vi "TOSA_MCS_Switch_Ray.vi"() -> ()   [LabVIEW 2012]
uses:
  <vilib>/DAQmx/create/channels.llb/DAQmx Create Channel (CO-Pulse Generation-Ticks).vi
  <vilib>/DAQmx/configure/timing.llb/DAQmx Timing (Implicit).vi
  <resource>/objmgr/daqmx.rc
  <vilib>/DAQmx/create/channels.llb/DAQmx Create Channel (DO-Digital Output).vi
panel:
  out "Error Out":errorcluster
  in  "stop 3":bool
  in  "Error In 3":errorcluster
  out "Error Out 3":errorcluster
  in  "Error In":errorcluster
  in  "Stop":bool
  in  "pulse count":u32=150 min=4 max=9000 step=2
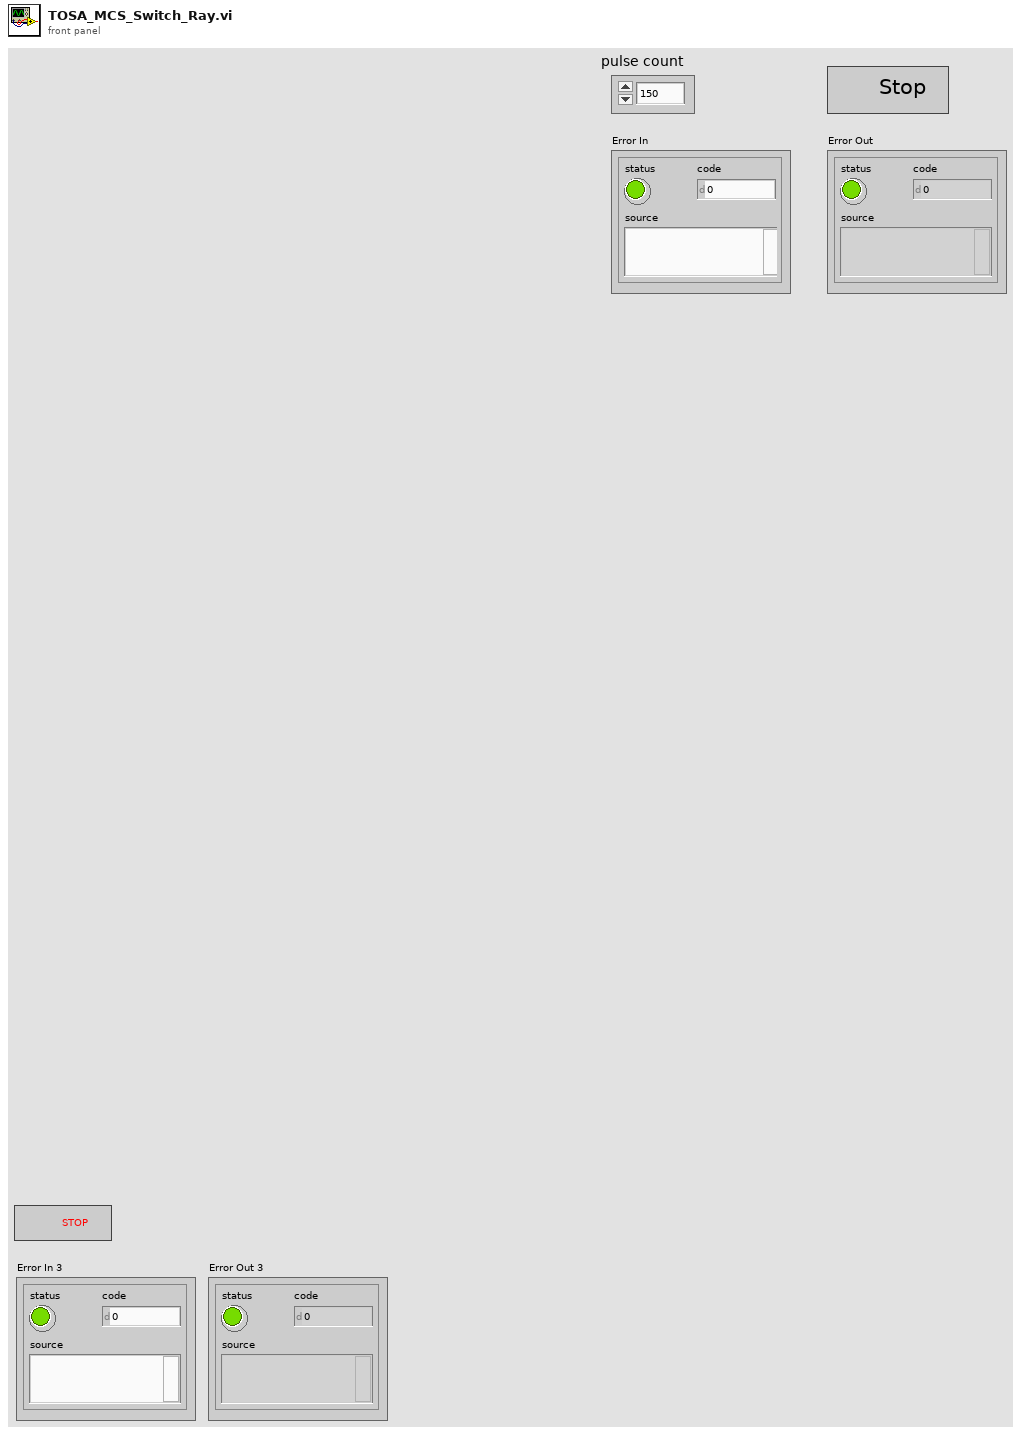
[diagram p1: front panel]
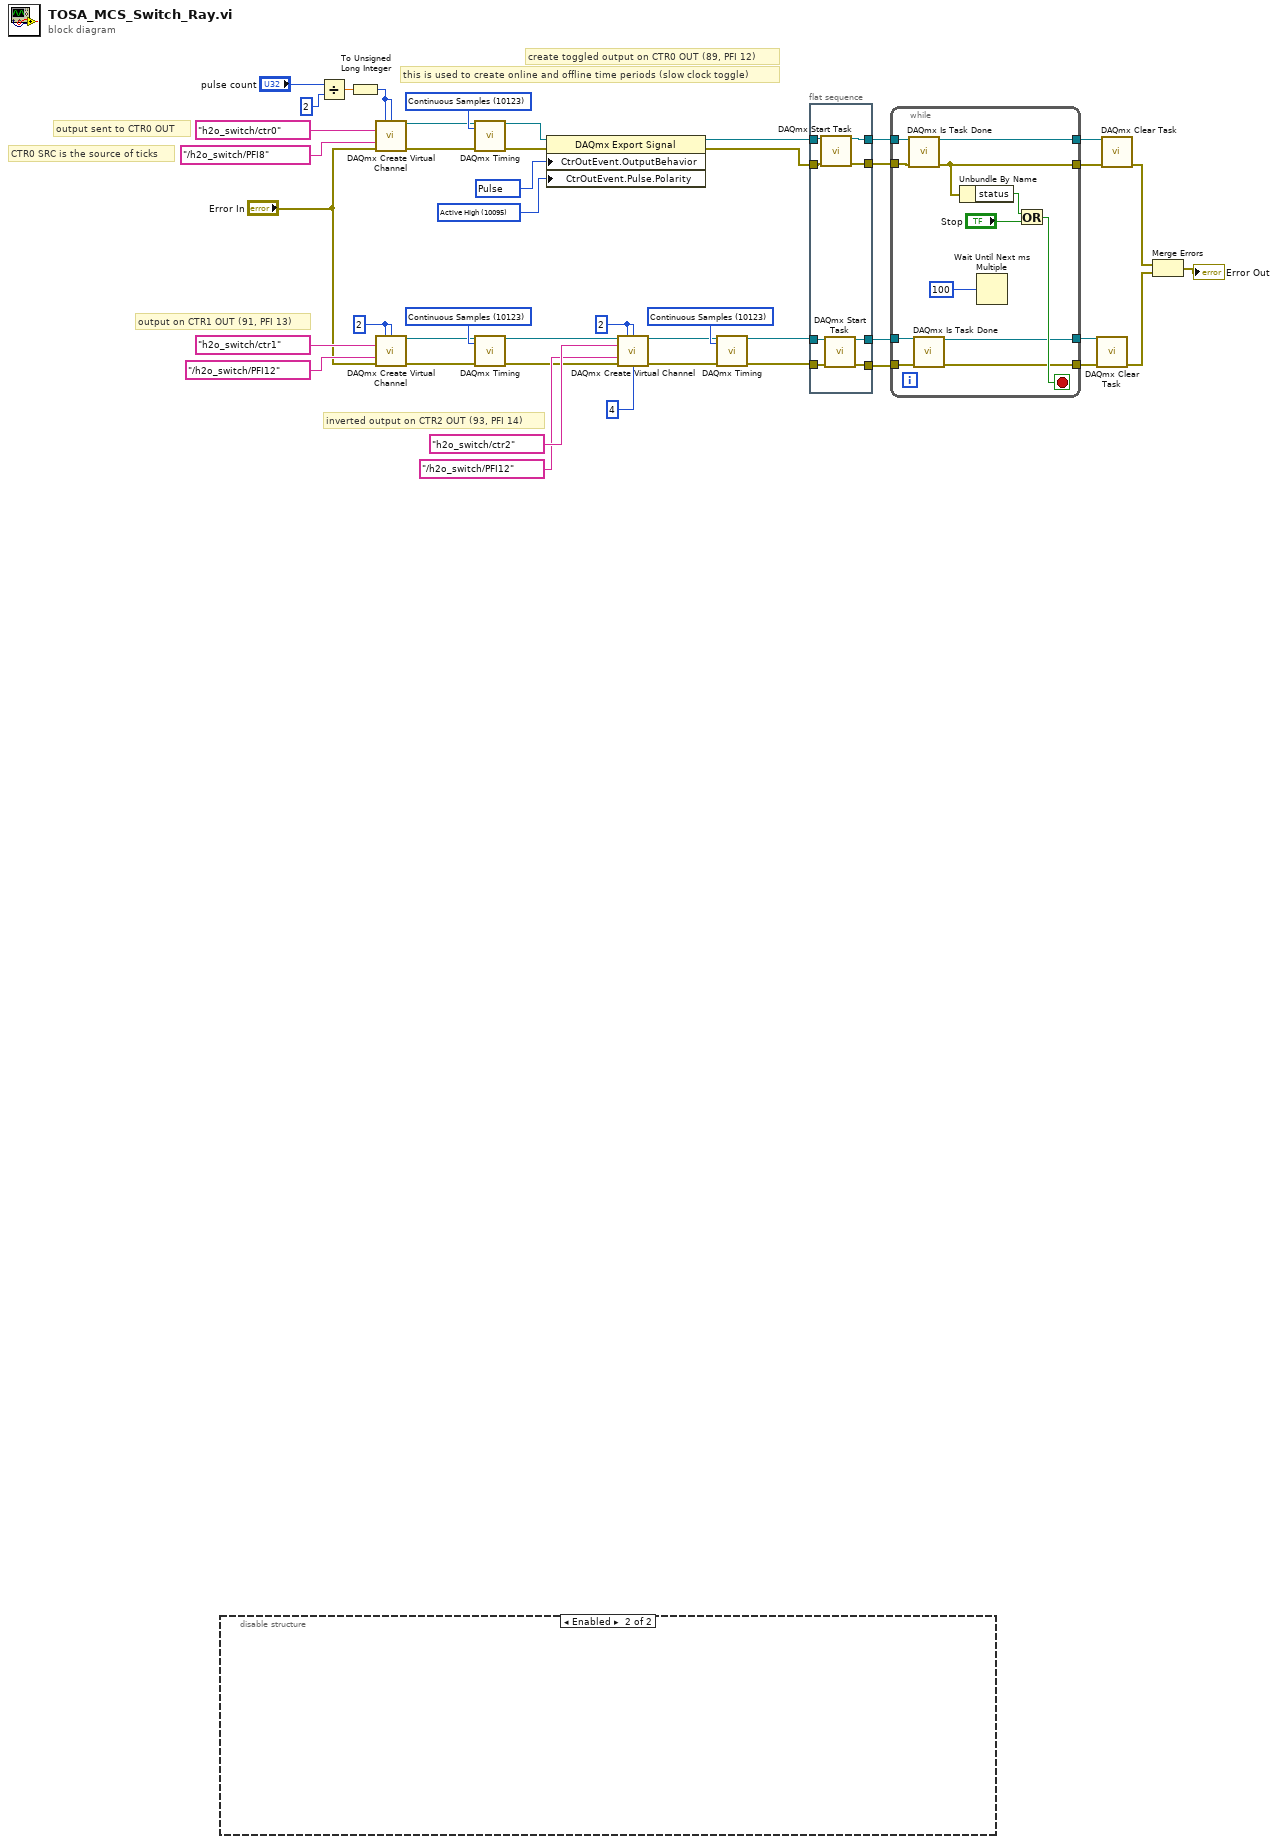
[diagram p0: block diagram]
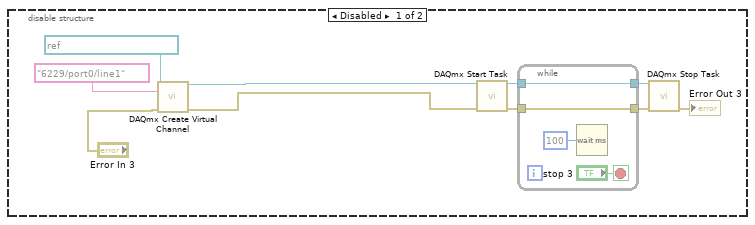
[diagram p2: hidden frame]
diagram:
  w18 = u32 2 ("high ticks")
  w23 = 10123 items=["Finite Samples"=10178, "Continuous Samples"=10123, "Hardware Timed Single Point"=12522] ("sample mode")
  w24 = u32 2 ("high ticks")
  w31 = 10123 items=["Finite Samples"=10178, "Continuous Samples"=10123, "Hardware Timed Single Point"=12522] ("sample mode")
  w32 = 10095 items=["Active High"=10095, "Active Low"=10096] ("CtrOutEvent.Pulse.Polarity")
  w44 = 10265 items=["Pulse"=10265, "Toggle"=10307] ("CtrOutEvent.OutputBehavior")
  w36 = 10123 items=["Finite Samples"=10178, "Continuous Samples"=10123, "Hardware Timed Single Point"=12522] ("sample mode")
  # "inverted output on CTR2 OUT (93, PFI 14)"
  # "output on CTR1 OUT (91, PFI 13)"
  # "output sent to CTR0 OUT"
  # "CTR0 SRC is the source of ticks"
  # "this is used to create online and offline time periods (slow clock toggle)"
  # "create toggled output on CTR0 OUT (89, PFI 12)"
  n1 = disable-structure shown="Enabled" {
    frame Disabled {
      n2 = call-poly <vilib>:"DAQmx Create Virtual Channel.vi"("task in"=refnum<k21> "MyDigitalOutTask_0", "lines"=tag "6229/port0/line1", "error in"="Error In 3") -> ("task out"=w47:refnum<k21>, "error out"=w46:errorcluster)  [unwired: 11 in]
      n3 = call <vilib>:"DAQmx Start Task.vi"("task/channels in"=w47, "error in"=w46) -> ("task out"=w50:refnum<k21>, "error out"=w51:errorcluster)  [unwired: 12 in]
      n4 = while {
        tunnel: w50 -> [w56]
        tunnel: w51 -> [w55]
        tunnel: [w56] -> w54
        tunnel: [w55] -> w53
        stop <- "stop 3" stop-if-true
        n5 = Wait (ms)(milliseconds to wait=u32 100) -> ()  [unwired: 1 out]
      }
      n6 = call <vilib>:"DAQmx Stop Task.vi"("task/channels in"=w54, "error in"=w53) -> ("error out"=→"Error Out 3":errorcluster)  [unwired: 12 in, 1 out]
    }
    frame Enabled {
    }
  }
  n7 = Divide(x="pulse count", y=u32 2) -> (x/y=w11:dbl)
  n8 = To Unsigned Long Integer(number=w11) -> (unsigned 32bit integer=w9:u32)
  n9 = call-poly <vilib>:"DAQmx Create Virtual Channel.vi"("high ticks"=w9, "low ticks"=w9, "counter"=tag "h2o_switch/ctr0", "source of ticks"=tag "/h2o_switch/PFI8", "error in"="Error In") -> ("task out"=w34:refnum<k21>, "error out"=w35:errorcluster)  [unwired: 9 in]
  n10 = call-poly <vilib>:"DAQmx Create Virtual Channel.vi"("high ticks"=w24, "low ticks"=w24, "counter"=tag "h2o_switch/ctr1", "source of ticks"=tag "/h2o_switch/PFI12", "error in"="Error In") -> ("task out"=w29:refnum<k21>, "error out"=w30:errorcluster)  [unwired: 9 in]
  n11 = call-poly <vilib>:"DAQmx Timing.vi"("task/channels in"=w34, "sample mode"=w36, "error in"=w35) -> ("task out"=w42:refnum<k21>, "error out"=w40:errorcluster)  [unwired: 11 in]
  n12 = call-poly <vilib>:"DAQmx Timing.vi"("task/channels in"=w29, "sample mode"=w31, "error in"=w30) -> ("task out"=w4:refnum<k21>, "error out"=w3:errorcluster)  [unwired: 11 in]
  n13 = property class="DAQmx Export Signal"(reference=w42, error in=w40, "CtrOutEvent.OutputBehavior"=w44, "CtrOutEvent.Pulse.Polarity"=w32) -> (reference out=w43:refnum<k21>, error out=w41:errorcluster)
  n14 = call-poly <vilib>:"DAQmx Create Virtual Channel.vi"("task in"=w4, "high ticks"=w18, "low ticks"=w18, "counter"=tag "h2o_switch/ctr2", "source of ticks"=tag "/h2o_switch/PFI12", "error in"=w3, "initial delay"=u32 4) -> ("task out"=w21:refnum<k21>, "error out"=w22:errorcluster)  [unwired: 7 in]
  n15 = call-poly <vilib>:"DAQmx Timing.vi"("task/channels in"=w21, "sample mode"=w23, "error in"=w22) -> ("task out"=w1:refnum<k21>, "error out"=w2:errorcluster)  [unwired: 11 in]
  n16 = flat-sequence {
    tunnel: [w64] -> w37
    tunnel: [w63] -> w33
    tunnel: [w62] -> w16
    tunnel: [w61] -> w15
    tunnel: w43 -> [w65]
    tunnel: w41 -> [w66]
    tunnel: w2 -> [w60]
    tunnel: w1 -> [w59]
    frame #0 {
      n17 = call <vilib>:"DAQmx Start Task.vi"("task/channels in"=w65, "error in"=w66) -> ("task out"=w64:refnum<k21>, "error out"=w63:errorcluster)  [unwired: 12 in]
      n18 = call <vilib>:"DAQmx Start Task.vi"("task/channels in"=w59, "error in"=w60) -> ("task out"=w62:refnum<k21>, "error out"=w61:errorcluster)  [unwired: 12 in]
    }
  }
  n19 = while {
    tunnel: w37 -> [w78]
    tunnel: w33 -> [w77]
    tunnel: [w74] -> w39
    tunnel: [w75] -> w38
    tunnel: w16 -> [w70]
    tunnel: w15 -> [w69]
    tunnel: [w68] -> w14
    tunnel: [w67] -> w13
    stop <- w76 stop-if-true
    n20 = call <vilib>:"DAQmx Is Task Done.vi"("task/channels in"=w78, "error in"=w77) -> ("task out"=w75:refnum<k21>, "error out"=w74:errorcluster)  [unwired: 11 in, 1 out]
    n21 = call <vilib>:"DAQmx Is Task Done.vi"("task/channels in"=w70, "error in"=w69) -> ("task out"=w68:refnum<k21>, "error out"=w67:errorcluster)  [unwired: 11 in, 1 out]
    n22 = Unbundle By Name(w74) -> ("status"=w73:bool)
    n23 = Wait Until Next ms Multiple(millisecond multiple=u32 100) -> ()  [unwired: 1 out]
    n24 = Or(x=w73, y="Stop") -> (x .or. y?=w76:bool)
  }
  n25 = call <vilib>:"DAQmx Clear Task.vi"("task in"=w14, "error in"=w13) -> ("error out"=w6:errorcluster)  [unwired: 13 in]
  n26 = call <vilib>:"DAQmx Clear Task.vi"("task in"=w38, "error in"=w39) -> ("error out"=w8:errorcluster)  [unwired: 13 in]
  n27 = Merge Errors(w8, w6) -> (→"Error Out":errorcluster)
